vi "ODMR sweep ACCES DAC control.vi"(8 "Save?":bool, 9 "file path (dialog if empty)":path=path "C:/Users/Ouyang Group/Documents/Data/5-13-15/ND Au 686 ODMR sweep 1", 10 "Freq Sweep Cluster":T1={"GPIB address 2"="19", "resolution (10 Hz:2) 2"=2, "band (1-26.5:2) 2"=2, "Freq max"=3300000000.0, "Start Freq"=5.5, "Voltage Step"=0.02, "rate"=100.0, "samples per channel"=500} {"rate" format="%0.2f"; "resolution (10 Hz:2) 2" items=["0.1 Hz", "1 Hz", "10 Hz", "100 Hz", "1 KHz", "10 KHz", "100 KHz", "1 MHz", "10 MHz", "100 MHz", "1 GHz"]}, 11 "Dot Tracking Cluster":T2={"RS232 settings"={"Portnumber"=6, "Baudrate"=5}, "X Parameters"={"Number of X Steps"=200, "Max X (V)"=2.0, "Min X (V)"=-2.0}, "Y Parameters"={"Number of Y Steps"=200, "Max Y (V)"=2.0, "Min Y (V)"=-2.0}, "X Pos"=97.0, "Y Pos"=112.0, "Z Pos"=52.78, "Tracking interval"=150.0} {"RS232 settings"."Portnumber" items=["COM1", "COM2", "COM3", "COM4", "COM5", "COM6", "COM7", "COM8", "COM9", "COM10", "COM11", "COM12", "COM13", "COM14", "COM15", "COM16", "COM17", "COM18", "COM19", "COM20", "COM21", "COM22", "COM23", "COM24", "COM25", "COM26", "COM27", "COM28", "COM29", "COM30"]; "RS232 settings"."Baudrate" items=["9600", "14400", "19200", "38400", "57600", "115200"]}) -> (0 "Z Position":dbl=31.0, 1 "Y Position":dbl=62.0, 2 "X Position":dbl=97.0, 3 "XY Graph":cluster{"Y":dbl[], "Y":dbl[]}[](graph), 4 "appended array":ext[][](array[numeric]))   [LabVIEW 2012]
uses:
  <vilib>/DAQmx/read.llb/DAQmx Read (Counter 1D DBL 1Chan NSamp).vi
  <vilib>/DAQmx/create/channels.llb/DAQmx Create Channel (CI-Count Edges).vi
  <vilib>/DAQmx/configure/timing.llb/DAQmx Timing (Sample Clock).vi
  <vilib>/DAQmx/miscellaneous.llb/DAQmx Fill In Error Info.vi
  <vilib>/Utility/file.llb/Write To Spreadsheet File (DBL).vi
  <vilib>/express/express arith-compare/Formula/XNode/ExpressFormulaBlockNode.xnode
  <resource>/objmgr/daqmx.rc
panel:
  in  "leveling file":path=path "C:/Users/Ouyang Group/Documents/Data/8-5-16/wavetek power calibration double sweep -4dbm interp 3"
  out "power":dbl
  out "voltage":dbl
  out "Frequency":dbl
  in  "stop":bool
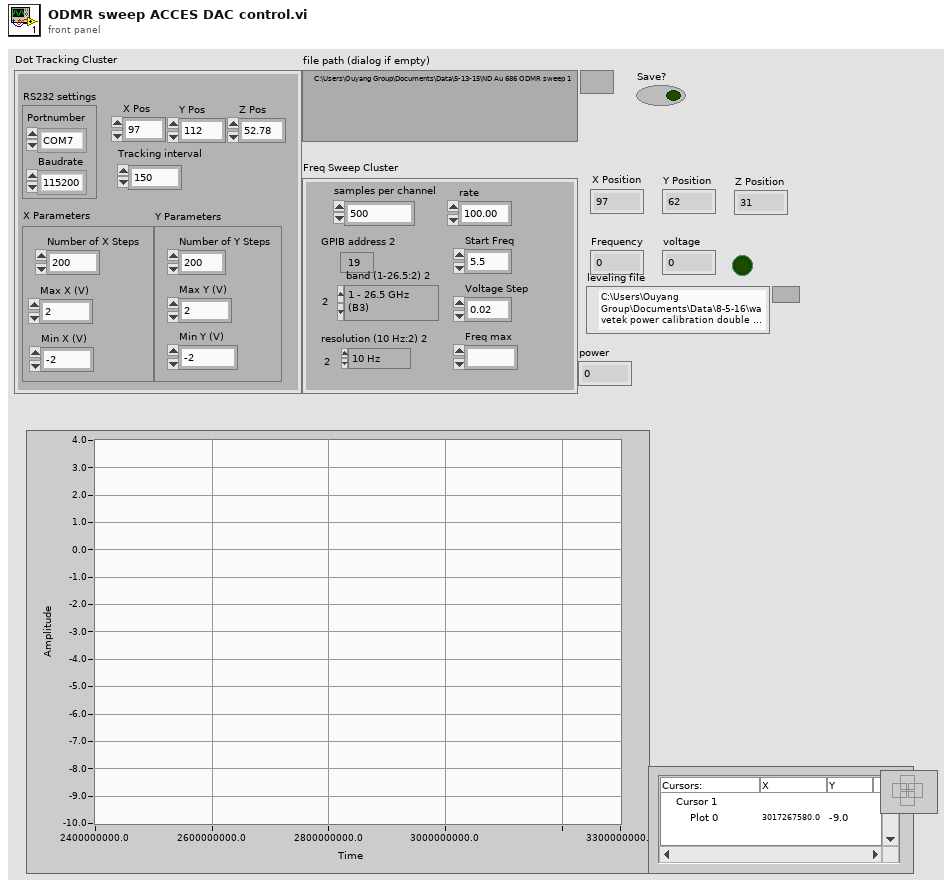
[diagram p1: front panel]
types:
  T1 = cluster{"GPIB address 2":string, "resolution (10 Hz:2) 2":i32, "band (1-26.5:2) 2":i32, "Freq max":ext, "Start Freq":dbl, "Voltage Step":dbl, "rate":dbl, "samples per channel":i32}
  T2 = cluster{"RS232 settings":cluster{"Portnumber":i32, "Baudrate":u16}, "X Parameters":cluster{"Number of X Steps":i32, "Max X (V)":dbl, "Min X (V)":dbl}, "Y Parameters":cluster{"Number of Y Steps":i32, "Max Y (V)":dbl, "Min Y (V)":dbl}, "X Pos":dbl, "Y Pos":dbl, "Z Pos":dbl, "Tracking interval":dbl}
  T3 = cluster{"Number of X Steps":i32, "Max X (V)":dbl, "Min X (V)":dbl}
  T4 = cluster{"Number of Y Steps":i32, "Max Y (V)":dbl, "Min Y (V)":dbl}
  T5 = cluster{"source lock":bool, "lock frequency (Hz)":ext, "coarse tune":bool}
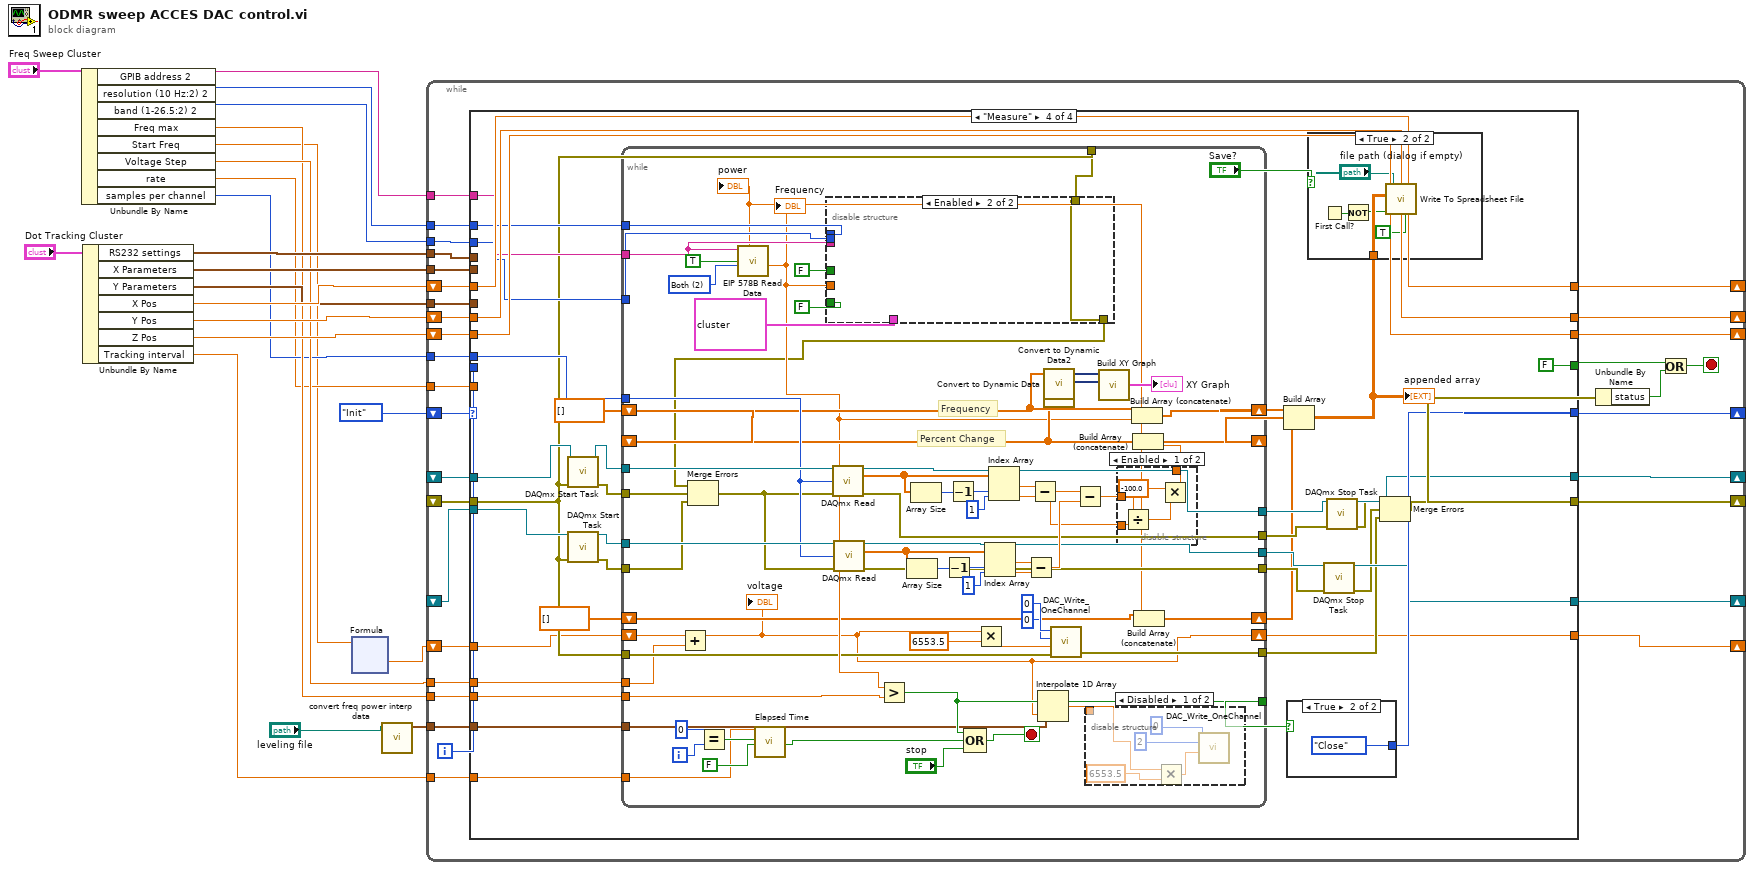
[diagram p0: block diagram]
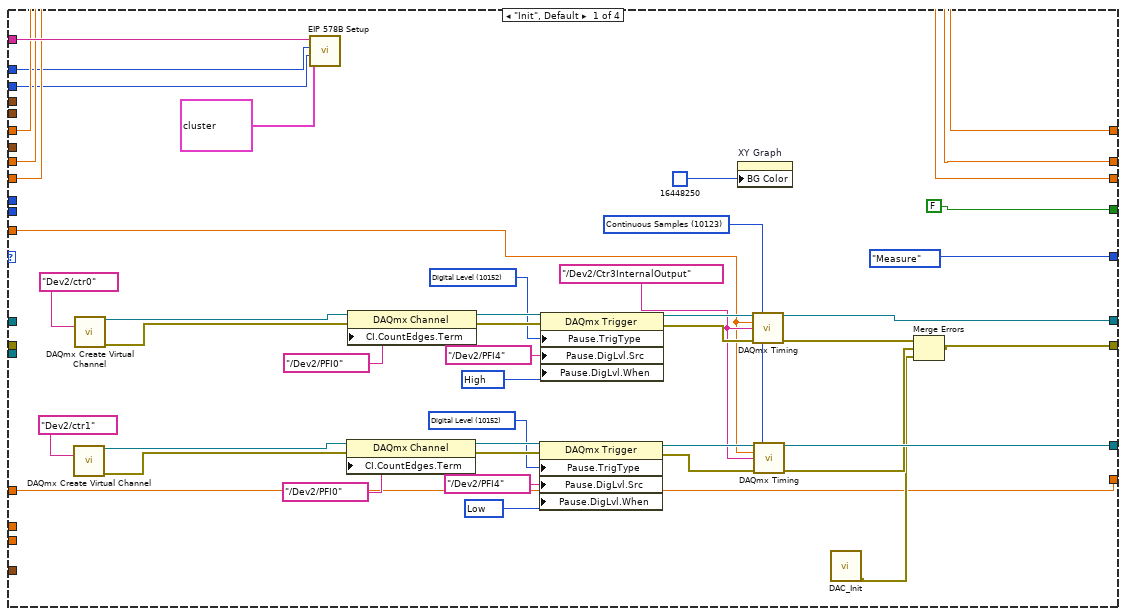
[diagram p2: hidden frame]
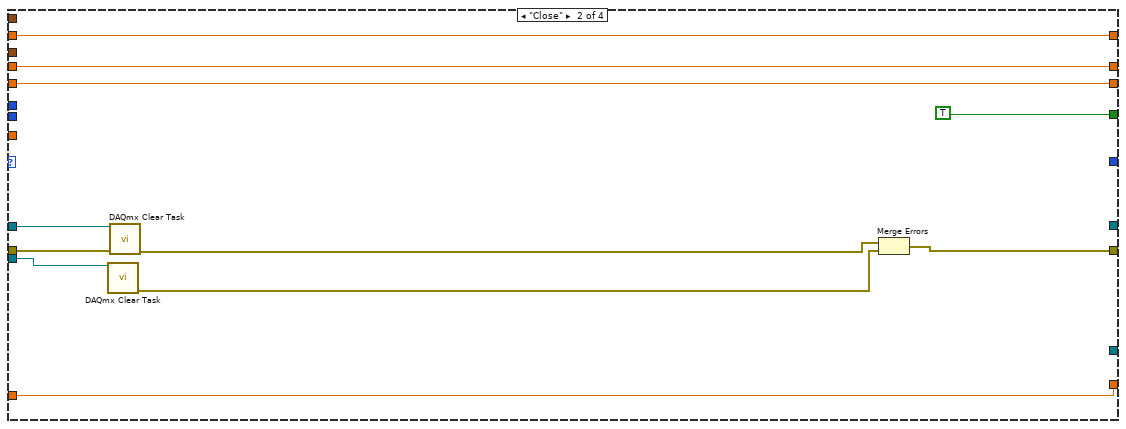
[diagram p3: hidden frame]
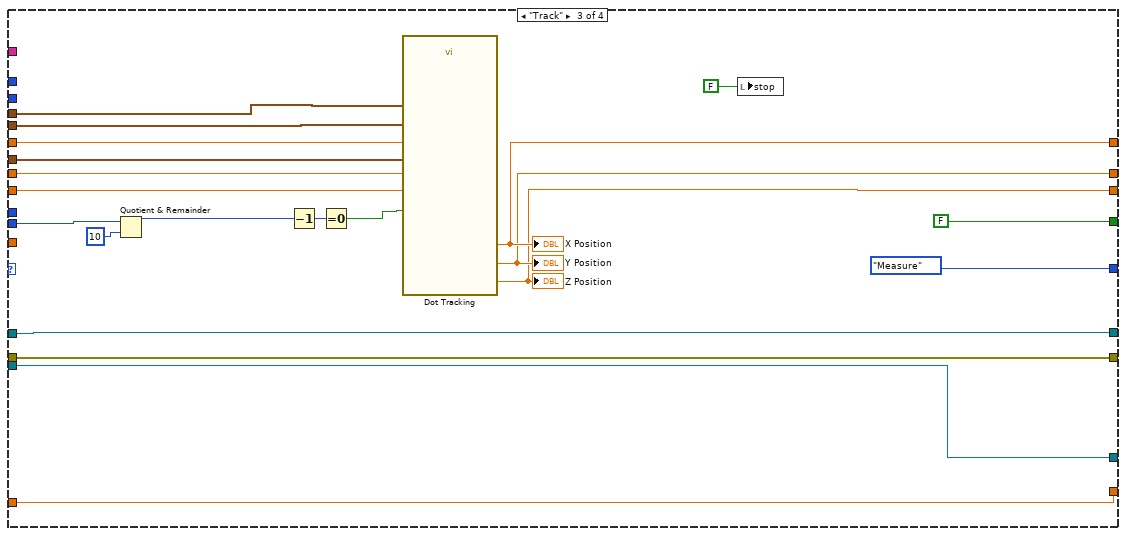
[diagram p4: hidden frame]
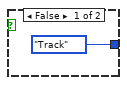
[diagram p6: hidden frame]
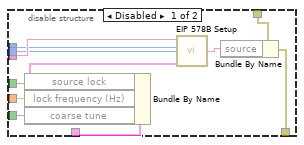
[diagram p9: hidden frame]
diagram:
  n1 = Unbundle By Name("Freq Sweep Cluster") -> ("GPIB address 2"=w11:string, "resolution (10 Hz:2) 2"=w10:i32, "band (1-26.5:2) 2"=w9:i32, "Freq max"=w7:ext, "Start Freq"=w3:dbl, "Voltage Step"=w8:dbl, "rate"=w5:dbl, "samples per channel"=w6:i32)
  n2 = Unbundle By Name("Dot Tracking Cluster") -> ("RS232 settings"=w16:cluster{"Portnumber":i32, "Baudrate":u16}, "X Parameters"=w15:T3, "Y Parameters"=w14:T4, "X Pos"=w19:dbl, "Y Pos"=w18:dbl, "Z Pos"=w17:dbl, "Tracking interval"=w13:dbl)
  n3 = xnode "Formula"("X1"=w3) -> ("Result"=w4:dbl)  [unwired: 1 in, 1 out]
  n4 = call "convert freq power interp data.vi"("file path (dialog if empty)"="leveling file") -> ("Array"=w1:cluster{dbl, dbl}[])  [unwired: 10 in]
  n5 = while {
    shift-right: [w49] -> _
    shift-left: enum16{"Init", "Measure", "Track", "Close"}."Init" -> [w53]
    tunnel: w11 -> [w52]
    shift-right: [w51] -> _
    shift-left: _ -> [w48]
    shift-right: [w50] -> _
    shift-left: _ -> [w47]
    shift-right: [w44] -> _
    shift-left: _ -> [w46]
    tunnel: w6 -> [w41]
    shift-right: [w36] -> _
    shift-left: w19 -> [w39]
    shift-right: [w35] -> _
    shift-left: w18 -> [w38]
    shift-right: [w34] -> _
    shift-left: w17 -> [w37]
    tunnel: w10 -> [w33]
    tunnel: w9 -> [w32]
    shift-right: [w29] -> _
    shift-left: w4 -> [w31]
    tunnel: w8 -> [w30]
    tunnel: w16 -> [w28]
    tunnel: w15 -> [w27]
    tunnel: w14 -> [w26]
    tunnel: w13 -> [w25]
    tunnel: w7 -> [w24]
    tunnel: w5 -> [w23]
    tunnel: w1 -> [w22]
    i -> [w45]
    stop <- w43 stop-if-true
    n6 = case shown="\"Measure\"" w53 {
      tunnel: [FALSE TRUE FALSE FALSE] -> w42
      tunnel: w52 -> [w94 _ _ w145]
      tunnel: [w69 _ w127 w157] -> w51
      tunnel: [w68 _ w126 w154] -> w50
      tunnel: [w65 w101 w120 w167] -> w44
      tunnel: [enum16{"Init", "Measure", "Track", "Close"}."Measure" _ enum16{"Init", "Measure", "Track", "Close"}."Measure" w166] -> w49
      tunnel: w48 -> [_ w105 w127 w163]
      tunnel: w47 -> [_ w103 w126 w160]
      tunnel: w46 -> [_ w104 w120 w140]
      tunnel: w45 -> [_ _ w121 _]
      tunnel: w41 -> [_ _ _ w150]
      tunnel: w39 -> [w61 w99 w116 w148]
      tunnel: w38 -> [w60 w98 w115 w147]
      tunnel: w37 -> [w59 w97 w114 w146]
      tunnel: [w61 w99 w113 w148] -> w36
      tunnel: [w60 w98 w112 w147] -> w35
      tunnel: [w59 w97 w111 w146] -> w34
      tunnel: w33 -> [w58 _ _ w144]
      tunnel: w32 -> [w57 _ _ w143]
      tunnel: w31 -> [w55 w96 w110 w138]
      tunnel: w30 -> [_ _ _ w137]
      tunnel: [w55 w96 w110 w136] -> w29
      tunnel: w28 -> [_ _ w109 _]
      tunnel: w27 -> [_ _ w108 _]
      tunnel: w26 -> [_ _ w107 _]
      tunnel: w25 -> [_ _ _ w135]
      tunnel: w24 -> [_ _ _ w134]
      tunnel: w23 -> [w54 _ _ _]
      tunnel: w22 -> [_ _ _ w128]
      frame "Init", Default {
        w70 = tag "/Dev2/Ctr3InternalOutput" ("source")
        w71 = 10123 items=["Finite Samples"=10178, "Continuous Samples"=10123, "Hardware Timed Single Point"=12522] ("sample mode")
        w76 = 10214 items=["High"=10192, "Low"=10214] ("Pause.DigLvl.When")
        w78 = 10152 items=["Analog Level"=10101, "Analog Window"=10103, "Digital Level"=10152, "Digital Pattern"=10398, "None"=10230] ("Pause.TrigType")
        w85 = 10192 items=["High"=10192, "Low"=10214] ("Pause.DigLvl.When")
        w87 = 10152 items=["Analog Level"=10101, "Analog Window"=10103, "Digital Level"=10152, "Digital Pattern"=10398, "None"=10230] ("Pause.TrigType")
        n7 = call-poly <vilib>:"DAQmx Create Virtual Channel.vi"("counter"=tag "Dev2/ctr1") -> ("task out"=w83:refnum<k21>, "error out"=w82:errorcluster)  [unwired: 13 in]
        n8 = call-poly <vilib>:"DAQmx Create Virtual Channel.vi"("counter"=tag "Dev2/ctr0") -> ("task out"=w92:refnum<k21>, "error out"=w91:errorcluster)  [unwired: 13 in]
        n9 = call "EIP 578B Setup.vi"("GPIB Address"=w94, "band (1-26.5 GHz:20)"=w58, "resolution (1 Hz:1)"=w57, "source locking"=T5 {"source lock"=FALSE, "lock frequency (Hz)"=1000000000.0, "coarse tune"=TRUE}) -> ()  [unwired: 2 in, 2 out]
        n10 = property class="DAQmx Channel"(reference=w83, error in=w82, "CI.CountEdges.Term"=tag "/Dev2/PFI0") -> (reference out=w80:refnum<k21>, error out=w79:errorcluster)
        n11 = property class="DAQmx Channel"(reference=w92, error in=w91, "CI.CountEdges.Term"=tag "/Dev2/PFI0") -> (reference out=w89:refnum<k21>, error out=w88:errorcluster)
        n12 = property class="DAQmx Trigger"(reference=w80, error in=w79, "Pause.TrigType"=w78, "Pause.DigLvl.Src"=tag "/Dev2/PFI4", "Pause.DigLvl.When"=w76) -> (reference out=w73:refnum<k21>, error out=w72:errorcluster)
        n13 = property class="DAQmx Trigger"(reference=w89, error in=w88, "Pause.TrigType"=w87, "Pause.DigLvl.Src"=tag "/Dev2/PFI4", "Pause.DigLvl.When"=w85) -> (reference out=w75:refnum<k21>, error out=w74:errorcluster)
        n14 = property on="XY Graph" class="XYGraph (strict)"("BG Color"=u32 16448250) -> ()  [unwired: 2 in, 2 out]
        n15 = call-poly <vilib>:"DAQmx Timing.vi"("task/channels in"=w75, "sample mode"=w71, "rate"=w54, "source"=w70, "error in"=w74) -> ("task out"=w69:refnum<k21>, "error out"=w67:errorcluster)  [unwired: 9 in]
        n16 = call-poly <vilib>:"DAQmx Timing.vi"("task/channels in"=w73, "sample mode"=w71, "rate"=w54, "source"=w70, "error in"=w72) -> ("task out"=w68:refnum<k21>, "error out"=w66:errorcluster)  [unwired: 9 in]
        n17 = call "DAC_Init.vi"() -> ("error out"=w56:errorcluster)  [unwired: 11 in]
        n18 = Merge Errors(w67, w66, w56) -> (w65:errorcluster)
      }
      frame "Close" {
        n19 = call <vilib>:"DAQmx Clear Task.vi"("task in"=w103) -> ("error out"=w102:errorcluster)  [unwired: 14 in]
        n20 = call <vilib>:"DAQmx Clear Task.vi"("task in"=w105, "error in"=w104) -> ("error out"=w100:errorcluster)  [unwired: 13 in]
        n21 = Merge Errors(w100, w102) -> (w101:errorcluster)
      }
      frame "Track" {
        n22 = Quotient & Remainder(x=w121, y=10) -> (x-y*floor(x/y)=w124:i32)  [unwired: 1 out]
        n23 = Decrement(x=w124) -> (x-1=w125:i32)
        n24 = Equal To 0?(x=w125) -> (x = 0?=w122:bool)
        n25 = call "Dot Tracking.vi"("X"=w108, "Y Parameters"=w107, "RS232 settings"=w109, "X Pos"=w116, "Y pos"=w115, "Z Pos"=w114, "Z-track?"=w122) -> ("X Position"=w113:dbl, "Y Position"=w112:dbl, "Z Position"=w111:dbl)  [unwired: 2 in, 4 out]
        "X Position" <- w113
        "Y Position" <- w112
        "Z Position" <- w111
        n26 = local write "stop"(FALSE ("stop")) -> ()
      }
      frame "Measure" {
        w149 = dbl[] []
        n27 = call <vilib>:"DAQmx Start Task.vi"("task/channels in"=w163, "error in"=w140) -> ("task out"=w161:refnum<k21>, "error out"=w162:errorcluster)  [unwired: 12 in]
        n28 = call <vilib>:"DAQmx Start Task.vi"("task/channels in"=w160, "error in"=w140) -> ("task out"=w159:refnum<k21>, "error out"=w158:errorcluster)  [unwired: 12 in]
        n29 = while {
          shift-right: [w229] -> w152
          shift-left: w149 -> [w216]
          shift-right: [w228] -> w132
          shift-left: w149 -> [w218]
          tunnel: w159 -> [w225]
          tunnel: [w224] -> w156
          tunnel: [w223] -> w165
          tunnel: [w220] -> w164
          tunnel: w162 -> [w222]
          tunnel: w161 -> [w221]
          tunnel: w158 -> [w194]
          tunnel: w150 -> [w219]
          tunnel: w145 -> [w206]
          tunnel: w144 -> [w205]
          tunnel: w143 -> [w204]
          tunnel: w140 -> [w196]
          tunnel: [w192] -> w142
          tunnel: [w191] -> w141
          tunnel: w140 -> [w188]
          tunnel: [w187] -> w139
          shift-right: [w177] -> w136
          shift-left: w138 -> [w186]
          tunnel: w137 -> [w185]
          tunnel: w135 -> [w182]
          tunnel: w134 -> [w181]
          shift-right: [w180] -> w129
          shift-left: dbl[] [] -> [w179]
          tunnel: w128 -> [w175]
          i -> [w208]
          stop <- w197 stop-if-true
          w212 = 2 items=["Frequency", "Power", "Both"] ("output mode (freq:0)")
          # "Percent Change"
          # "Frequency"
          n30 = Add(x=w186, y=w185) -> (x+y=w177:dbl)
          "voltage" <- w177
          n31 = Equal?(x=0, y=w208) -> (x = y?=w207:bool)
          n32 = call "EIP 578B Read Data.vi"("output mode (freq:0)"=w212, "fast (T=active)"=TRUE, "GPIB"=w206) -> ("Power (dBm)"=w176:ext, "frequency (Hz)"=w200:ext)  [unwired: 1 in, 2 out]
          "Frequency" <- w200
          "power" <- w176
          n33 = call "Elapsed Time"("Time Target (s)"=w182, "Reset"=w207, "Auto Reset"=FALSE) -> ("Time has Elapsed"=w199:bool)  [unwired: 9 in, 7 out]
          n34 = disable-structure shown="Enabled" {
            disable-tunnel: w206 -> [w264 _]
            disable-tunnel: w205 -> [w263 _]
            disable-tunnel: w204 -> [w262 _]
            disable-tunnel: T5 {"source lock"=FALSE, "lock frequency (Hz)"=1000000000.0, "coarse tune"=TRUE} ("source locking") -> [w261 _]
            disable-tunnel: FALSE ("source lock") -> [w260 _]
            disable-tunnel: FALSE ("coarse tune") -> [w259 _]
            disable-tunnel: w200 -> [w257 _]
            disable-tunnel: w196 -> [w256 w265]
            disable-tunnel: [w254 w265] -> w195
            frame Disabled {
              n35 = Bundle By Name(cluster=w261, "source lock"=w260, "lock frequency (Hz)"=w257, "coarse tune"=w259) -> (w258:T5)
              n36 = call "EIP 578B Setup.vi"("GPIB Address"=w264, "band (1-26.5 GHz:20)"=w263, "resolution (1 Hz:1)"=w262, "source locking"=w258) -> ("status messages"=w255:string)  [unwired: 2 in, 1 out]
              n37 = Bundle By Name(cluster=w256, "source"=w255) -> (w254:errorcluster)
            }
            frame Enabled {
            }
          }
          n38 = Merge Errors(w195, w222, w194) -> (w193:errorcluster)
          n39 = call-poly <vilib>:"DAQmx Read.vi"("task/channels in"=w221, "number of samples per channel"=w219, "error in"=w193) -> ("task out"=w223:refnum<k21>, "data"=w242:dbl[], "error out"=w224:errorcluster)  [unwired: 10 in]
          n40 = call-poly <vilib>:"DAQmx Read.vi"("task/channels in"=w225, "number of samples per channel"=w219, "error in"=w193) -> ("task out"=w220:refnum<k21>, "data"=w231:dbl[], "error out"=w191:errorcluster)  [unwired: 10 in]
          n41 = Greater?(x=w200, y=w181) -> (0:w192:bool)
          n42 = Array Size(array=w231) -> (size(s)=w236:i32)
          n43 = Array Size(array=w242) -> (size(s)=w241:i32)
          n44 = Decrement(x=w236) -> (x-1=w235:i32)
          n45 = Decrement(x=w241) -> (x-1=w240:i32)
          n46 = Compound Arithmetic op=OR(w192, w199, "stop") -> (w197:bool)
          n47 = Multiply(x=w177, y=6553.5) -> (x*y=w184:dbl)
          n48 = Index Array(array=w231, index #1=w235, index #2=1 ("index")) -> (element #1=w232:dbl, element #2=w233:dbl)
          n49 = Index Array(array=w242, index #1=w240, index #2=1 ("index")) -> (element #1=w237:dbl, element #2=w238:dbl)
          n50 = Subtract(x=w232, y=w233) -> (x-y=w230:dbl)
          n51 = Subtract(x=w237, y=w238) -> (x-y=w226:dbl)
          n52 = Interpolate 1D Array(1:w177, 2:w175) -> (0:w178:dbl)
          n53 = call "Convert to Dynamic Data"("Array"=w218) -> ("Dynamic Data Type"=w217:dynamicdata)  [unwired: 3 in]
          n54 = call "Convert to Dynamic Data2"("Array"=w216) -> ("Dynamic Data Type"=w215:dynamicdata)  [unwired: 3 in]
          n55 = call "DAC_Write_OneChannel.vi"("error in (no error)"=w188, "Value"=w184, "Channel"=u16 0, "DeviceIndex"=u64 0) -> ("error out"=w187:errorcluster)  [unwired: 6 in, 1 out]
          n56 = Subtract(x=w226, y=w230) -> (x-y=w227:dbl)
          n57 = disable-structure shown="Disabled" {
            disable-tunnel: w178 -> [w243 _]
            frame Disabled {
              n58 = Multiply(x=w243, y=6553.5) -> (x*y=w246:dbl)
              n59 = call "DAC_Write_OneChannel.vi"("Value"=w246, "Channel"=u16 2, "DeviceIndex"=u64 0) -> ()  [unwired: 7 in, 2 out]
            }
            frame Enabled {
            }
          }
          n60 = call "Build XY Graph"("Y Input"=w215, "X Input"=w217) -> ("XY Graph"=→"XY Graph":cluster{"Y":dbl[], "Y":dbl[]}[])  [unwired: 3 in, 6 out]
          n61 = disable-structure shown="Enabled" {
            disable-tunnel: w227 -> [w252 w253]
            disable-tunnel: w226 -> [w251 _]
            disable-tunnel: [w249 w253] -> w213
            frame Enabled {
              n62 = Divide(x=w252, y=w251) -> (x/y=w250:dbl)
              n63 = Multiply(x=-100.0, y=w250) -> (x*y=w249:dbl)
            }
            frame Disabled {
            }
          }
          n64 = Build Array (concatenate)(w218, w200) -> (w228:ext[])
          n65 = Build Array (concatenate)(w216, w213) -> (w229:dbl[])
          n66 = Build Array (concatenate)(w179, w176) -> (w180:ext[])
        }
        n67 = Build Array(w132, w152, w129) -> (w151:ext[][])
        "appended array" <- w151
        n68 = case shown="True" w142 {
          tunnel: [enum16{"Init", "Measure", "Track", "Close"}."Track" enum16{"Init", "Measure", "Track", "Close"}."Close"] -> w166
          frame False {
          }
          frame True {
          }
        }
        n69 = case shown="True" "Save?" {
          tunnel: w151 -> [_ w172]
          frame False {
          }
          frame True {
            n70 = First Call?() -> (First Call?: T/F=w171:bool)
            n71 = Not(x=w171) -> (.not. x?=w170:bool)
            n72 = call-poly <vilib>:"Write To Spreadsheet File.vi"("transpose? (no:F)"=TRUE, "append to file? (new file:F)"=w170, "2D data"=w172, "file path (dialog if empty)"="file path (dialog if empty)") -> ()  [unwired: 4 in, 1 out]
          }
        }
        n73 = call <vilib>:"DAQmx Stop Task.vi"("task/channels in"=w164, "error in"=w141) -> ("task out"=w154:refnum<k21>, "error out"=w153:errorcluster)  [unwired: 12 in]
        n74 = call <vilib>:"DAQmx Stop Task.vi"("task/channels in"=w165, "error in"=w156) -> ("task out"=w157:refnum<k21>, "error out"=w155:errorcluster)  [unwired: 12 in]
        n75 = Merge Errors(w155, w153, w139) -> (w167:errorcluster)
      }
    }
    n76 = Unbundle By Name(w44) -> ("status"=w40:bool)
    n77 = Or(x=w42, y=w40) -> (x .or. y?=w43:bool)
  }
